vi "stateMachine.vi"() -> ()   [LabVIEW 2014]
uses:
  <vilib>/dex/Stream Element Allocation Mode.ctl
  <vilib>/Platform/TimedLoop/XDataNode/wakeup.ctl
  <vilib>/Platform/TimedLoop/XDataNode/XDNodeRunTimeDep.lvlib
  <vilib>/Platform/TimedLoop/XDataNode/nitl_modes.ctl
  <vilib>/Platform/TimedLoop/XDataNode/timing_clust.ctl
  <vilib>/platform/TimedLoop/XDataNode/XDataNode.xnode
  <resource>/objmgr/ni.dex.rc
  UDP_Para_def.ctl
  <vilib>/DAQmx/write.llb/DAQmx Write (Digital 1D Bool NChan 1Samp 1Line).vi
  states_def.ctl
  daq_channel_read_parameter.ctl
panel:
  out "rightcounter":i32
  out "leftcounter":i32
  out "beh type":string
  out "vs type":string
  out "Tab Control":enum32{"State Machine"}(tab)
  in  "vsFilterPeriod_uS":i32=500 format="%#1.6f"
  in  "lickThreshold_V":fxp<+/-,16,5> format="%#.4g"
  in  "vsThreshold_V":fxp<+/-,16,5> format="%#.4g"
  in  "audioThreshold_V":fxp<+/-,16,5> format="%#.4g"
  in  "audioFilterPeriod_uS":i32=50000 format="%#1.6f"
  in  "audioOffState_V":fxp<+/-,16,5> format="%#.4g"
  out "rtFIFOsize":u32=50
  out "rtFIFOtimeout":u32
  out "rtFIFOdataPool":u32=50
  out "stateMachineCycle_uS":i64=500
  out "(Actual)":i64
  in  "delay_uS":u32
  out "IP_RT":string="192.168.137.2"
  in  "port_broadcast":u16=9091
  out "IP_host":string="192.168.137.1"
  out "port_host":u16=9090
  in  "Tab Control 2":enum32{"Data Transfer"}(tab)
  out "stream counter":u32
  out "Is Connected":bool
  out "Available Elements for Writing":i32
  out "stream writer buffer size":i32=500
  in  "rewardPeriod_uS":u32
  in  "waterOn_uS":u32
  in  "timeout_uS":u32=5000000
  in  "shockOn_uS":u32
  in  "Stop state":bool
  out "Initial data received":bool
  out "Tab Control 3":enum32{"Current status"}(tab)
  in  "toneReward":bool
  out "ABORT":bool
  out "trialStart":bool
  out "trialDone":bool
  out "Busy":bool
  out "stateLatched":bool
  out "curKey":u32=1
  out "curState":u32
  out "rtFIFOdataDim":i32
  in  "manualShock":bool
  in  "manualWaterRight":bool
  in  "manualWaterLeft":bool
  in  "lickReward":bool
  in  "allowPunish":bool
  in  "forceLRswitch":bool
  in  "allowCorrection":bool
  in  "allowAutoWater":bool
  out "error out":errorcluster
  in  "trialKey":i32[](array[numeric])
  in  "rwdrefPeriod_uS":u32
  out "FlagWaterLeft":bool
  in  "chanellParaCluster":T1={"audioOffState_V"=0.0, "audioFilterPeriod_uS"=50000, "audioThreshold_V"=0.0, "vsThreshold_V"=0.0, "vsFilterPeriod_uS"=0, "lickThreshold_V"=0.0} {"vsFilterPeriod_uS" format="%#1.6f"; "audioFilterPeriod_uS" format="%#1.6f"}
  out "leftWaterOnFlag":bool
  out "rightWaterOnFlag":bool
  out "contNoReward":i32
  out "rewardStatus":bool
types:
  T1 = typedef "daq_channel_read_parameter.ctl" = cluster{"audioOffState_V":fxp<+/-,16,5>, "audioFilterPeriod_uS":i32, "audioThreshold_V":fxp<+/-,16,5>, "vsThreshold_V":fxp<+/-,16,5>, "vsFilterPeriod_uS":i32, "lickThreshold_V":fxp<+/-,16,5>}
  T2 = typedef "XDNodeRunTimeDep.lvlib/timing_clust.ctl" = cluster{"Expected End [f-1]":u64, "Actual End [f-1]":u64, "Finished Late? [f-1]":bool, "Expected End [i-1]":u64, "Actual End [i-1]":u64, "Finished Late? [i-1]":bool, "Expected Start [i]":u64, "Actual Start [i]":u64, "Expected Start [f]":u64, "Actual Start [f]":u64, "Source Name":string, "Structure Name":string, "Period":i64, "Deadline":i64, "Offset":i64, "Start":i64, "Priority":i32, "Timeout":i32, "Mode":T3, "Wakeup Reason":T4, "Error":errorcluster, "Source Type":string, "Secondary Source Type":string, "Global End Time":u64, "Global Start Time":u64, "Frame Duration":u64, "Iteration Duration":u64, "Assigned CPU":i32, "I/O Scan Engine Mode":u32}
  T3 = typedef "XDNodeRunTimeDep.lvlib/nitl_modes.ctl" = enum32{"No Change", "Process missed periods, maintain original phase", "Discard missed periods, maintain original phase", "Process missed periods, ignore original phase", "Discard missed periods, ignore original phase"}
  T4 = typedef "XDNodeRunTimeDep.lvlib/wakeup.ctl" = enum32{"Normal", "Aborted", "Asynchronous wakeup", "Timing source error", "Timed loop error", "Timeout"}
  T5 = typedef "states_def.ctl" = enum16{"idle", "vs before", "vs", "vs after", "delay", "tone before", "tone", "tone after", "cycle end", "reward", "reward refractory", "punish", "punish refractory", "timeout", "exit", "manualwater"}
  T6 = typedef "Stream Element Allocation Mode.ctl" = u32
  T7 = typedef "UDP_Para_def.ctl" = enum16{"no", "start", "stop", "dly", "rwp", "rwf", "wdr", "shd", "tod", "lkr", "tlr", "alp", "msh", "mwl", "mwr", "lth", "vth", "ath", "aof", "afp", "vfp"}
  T8 = cluster{"leftLick":bool, "rightLick":bool, "visualStimuli2":bool, "tone":bool, "visualStimuli1":bool}
  T9 = cluster{"leftLick":dbl, "rightLick":dbl, "visualStimuli2":dbl, "tone":dbl, "visualStimuli1":dbl}
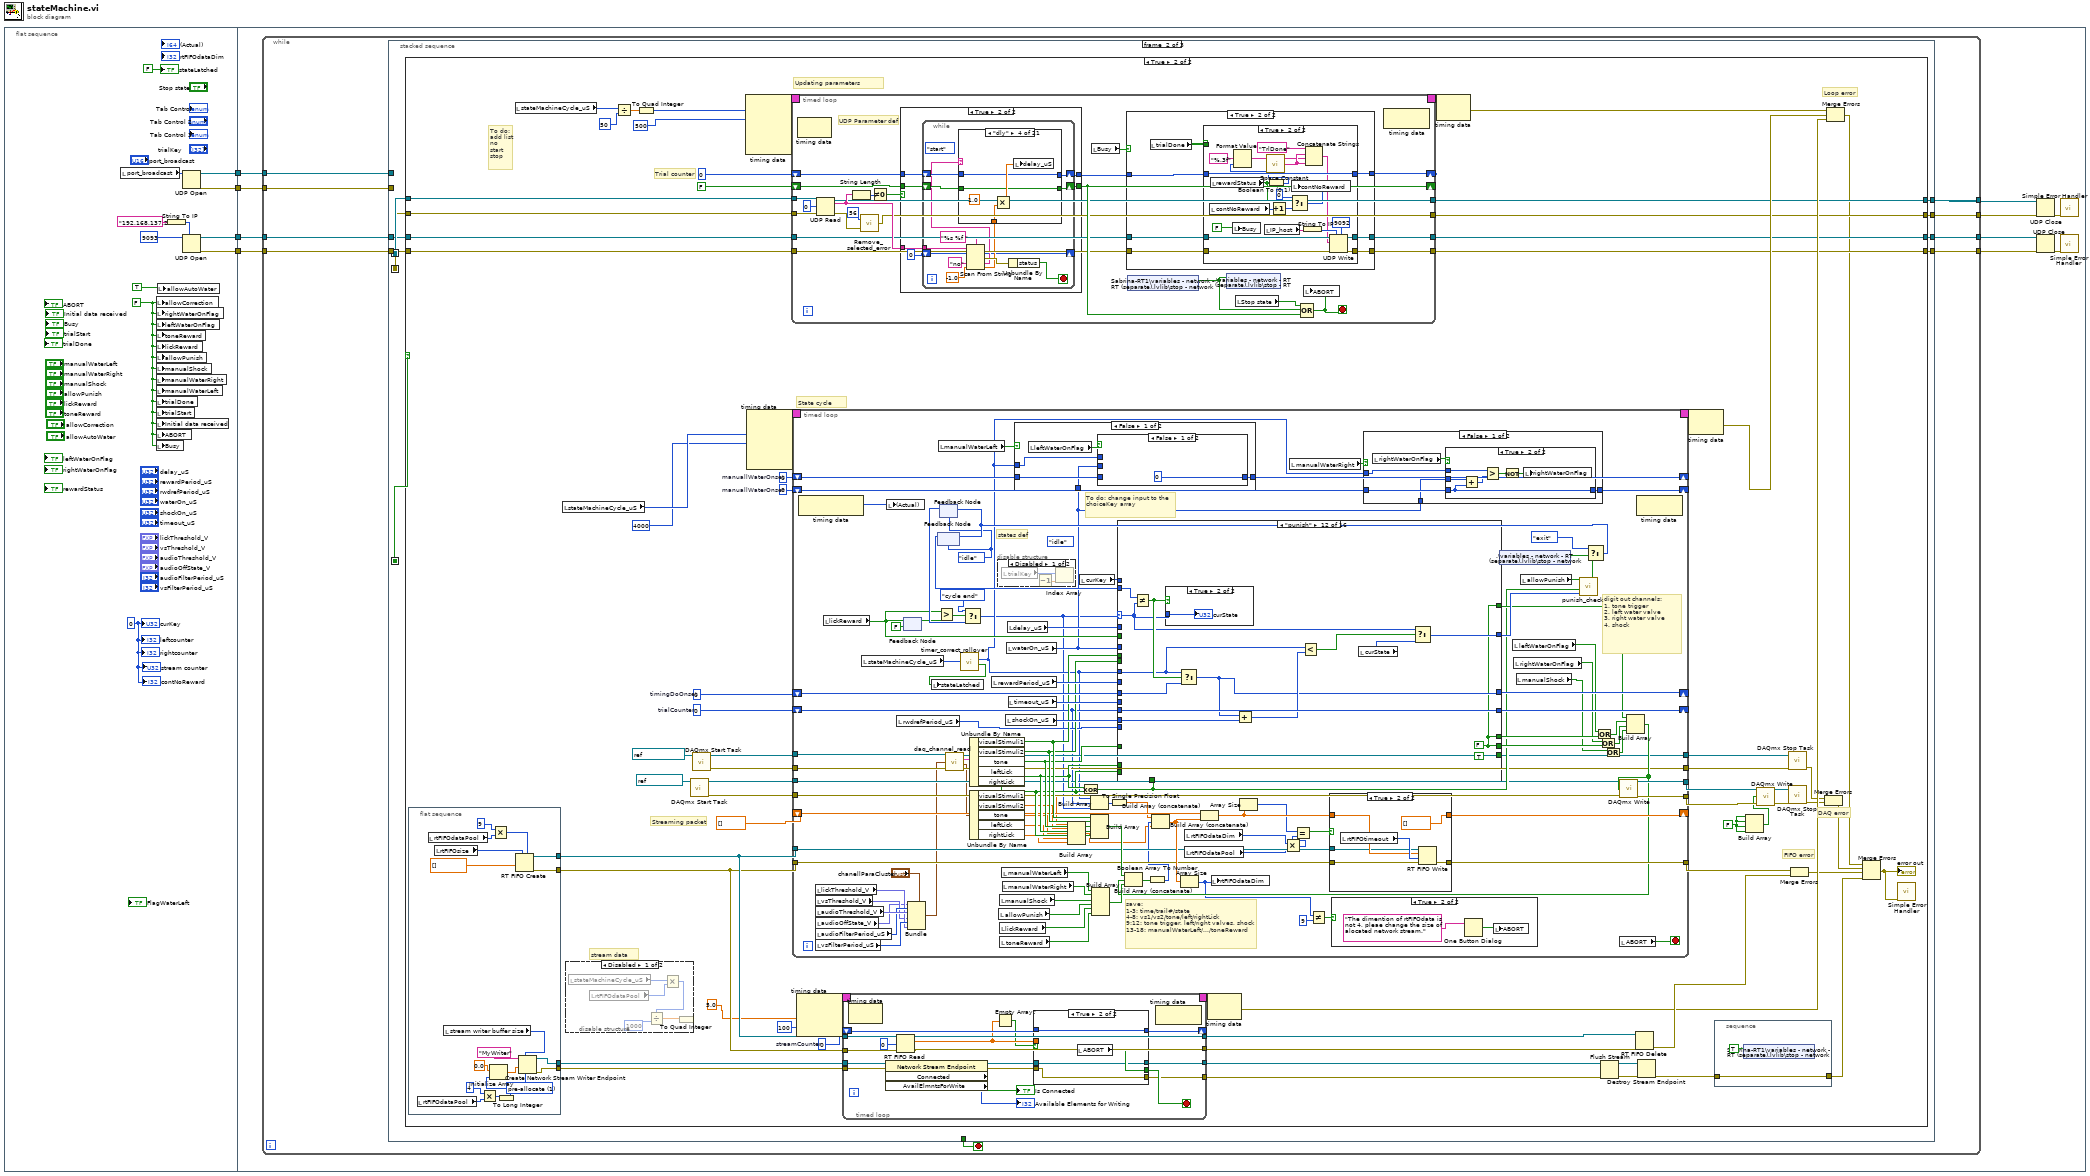
[diagram p0: block diagram]
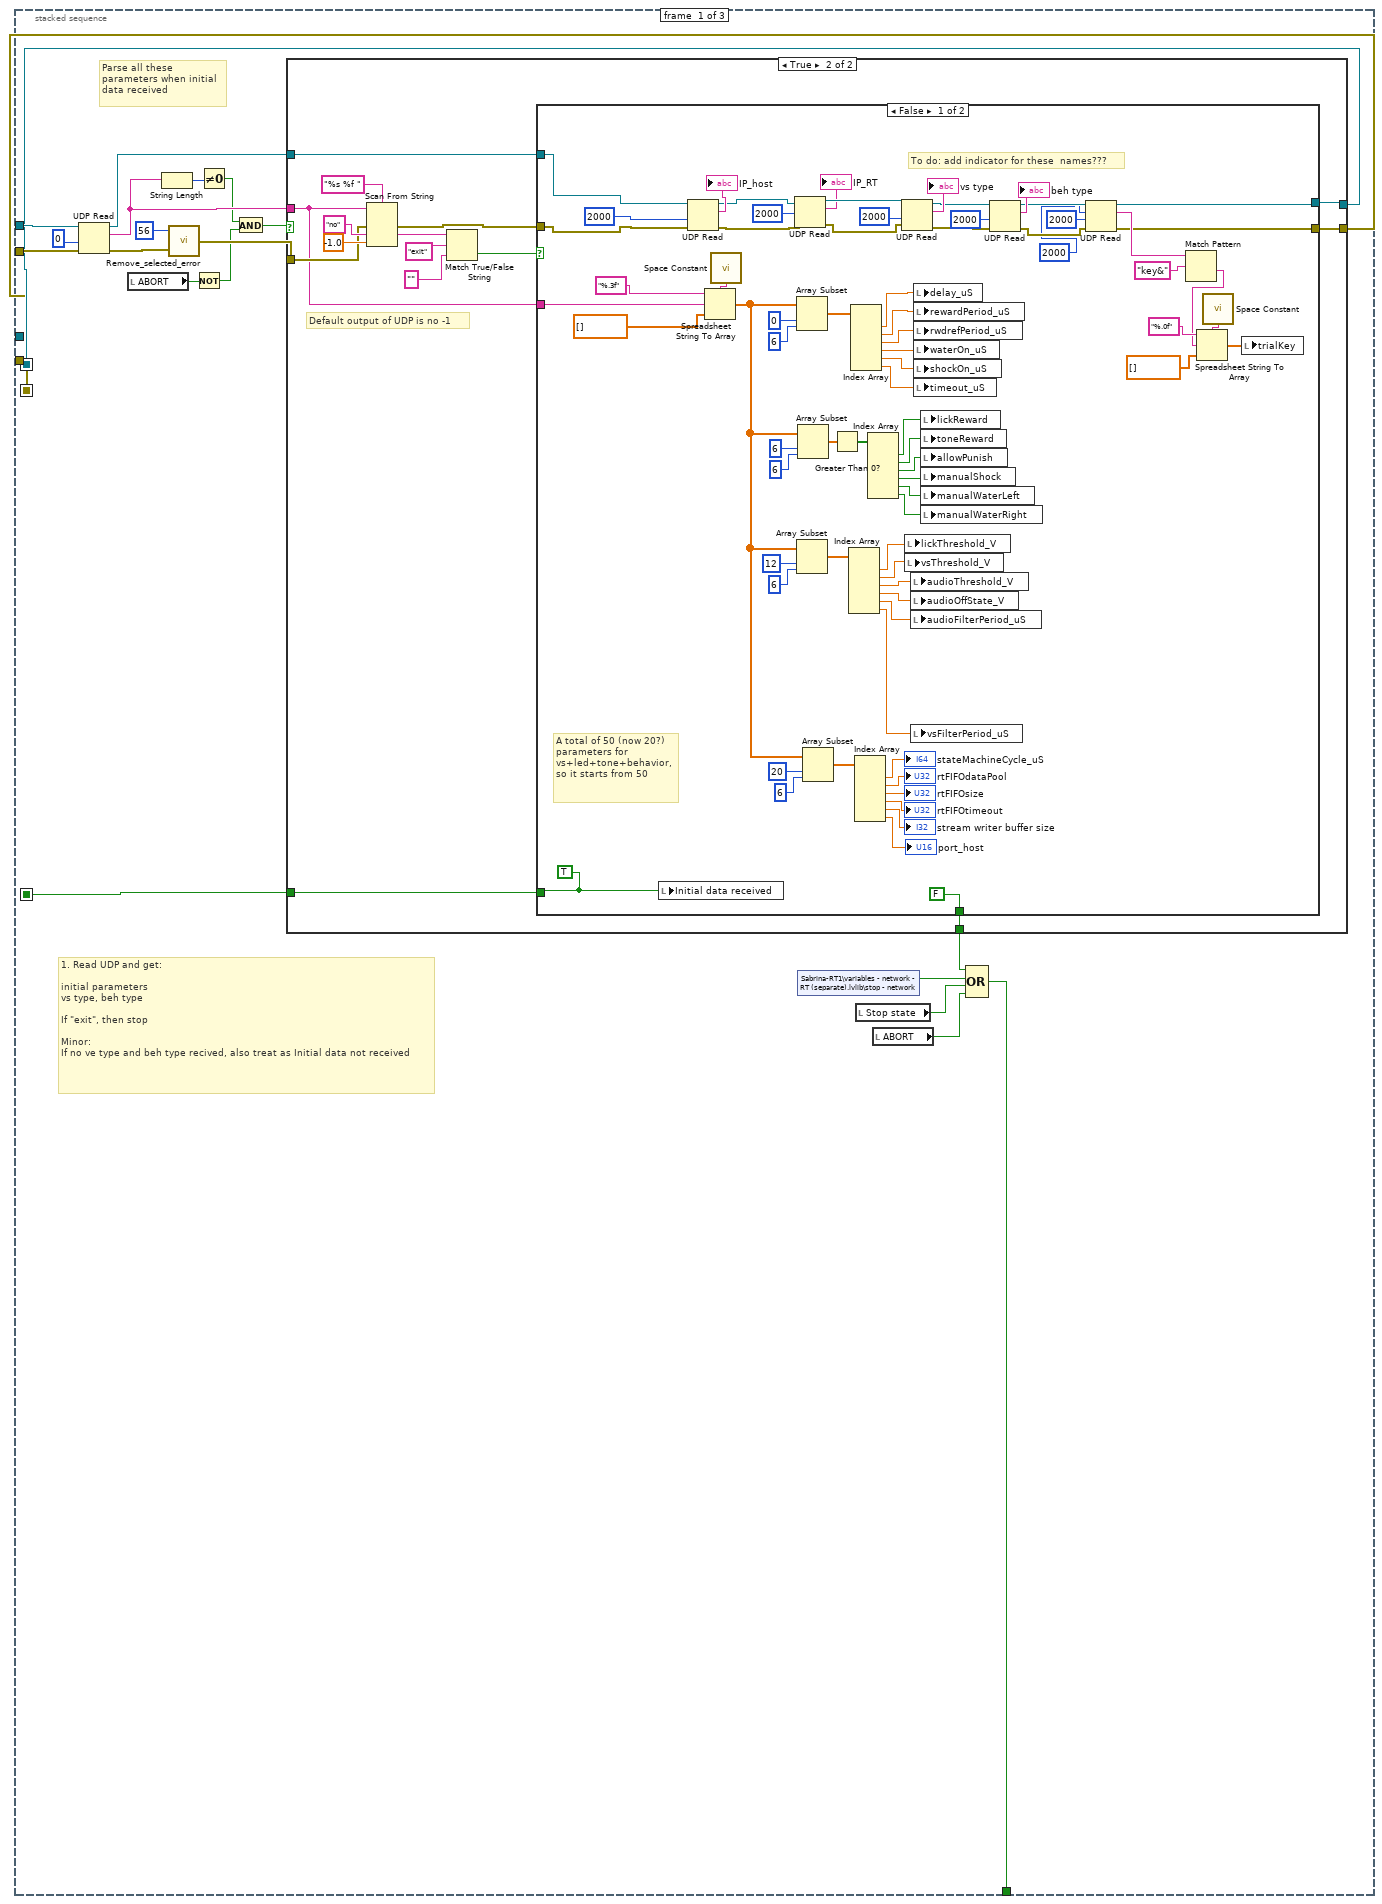
[diagram p2: hidden frame]
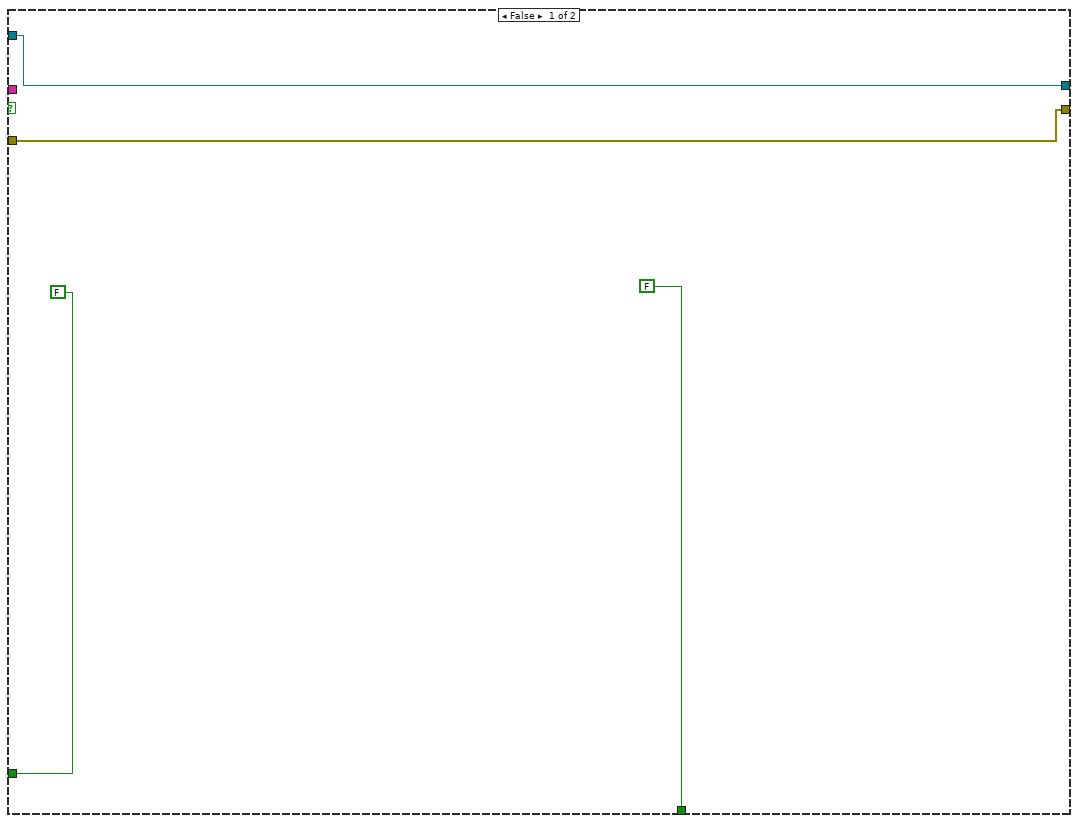
[diagram p3: hidden frame]
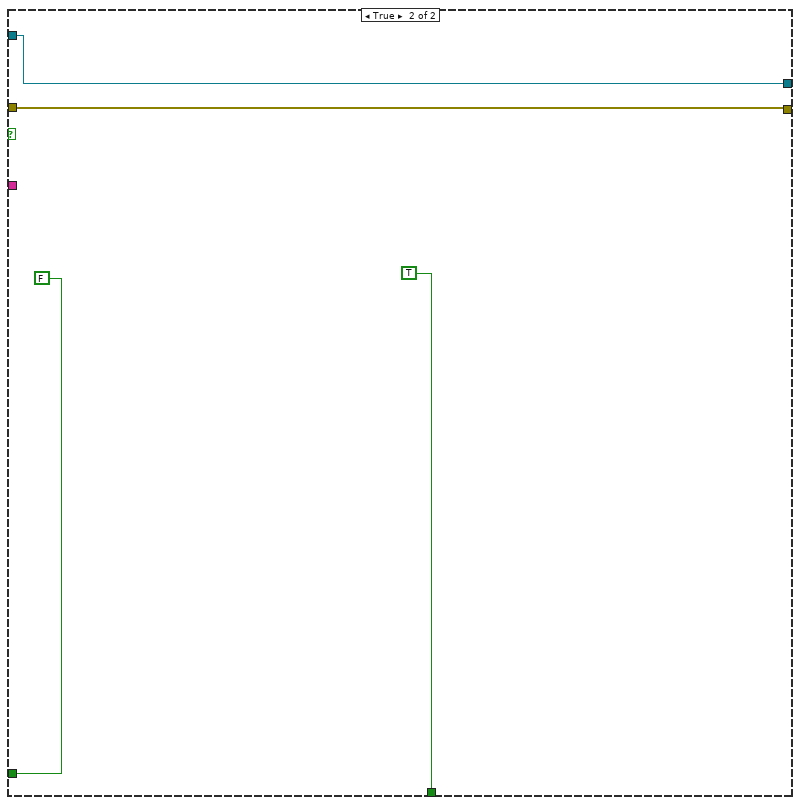
[diagram p4: hidden frame]
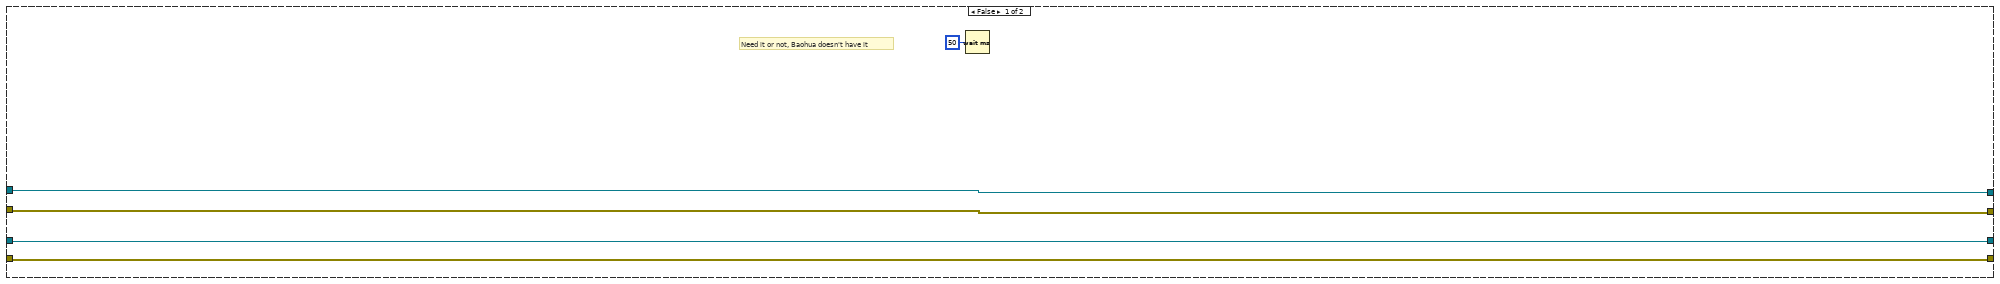
[diagram p5: hidden frame]
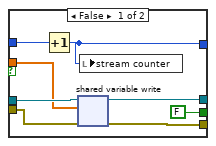
[diagram p7: hidden frame]
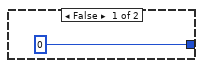
[diagram p9: hidden frame]
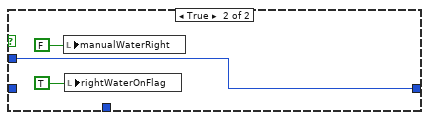
[diagram p10: hidden frame]
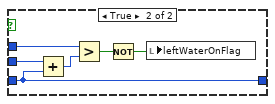
[diagram p11: hidden frame]
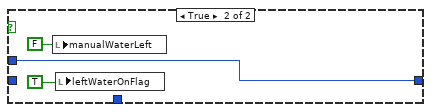
[diagram p12: hidden frame]
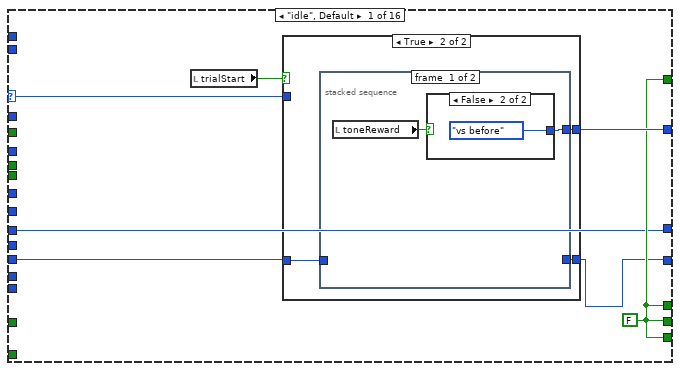
[diagram p15: hidden frame]
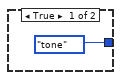
[diagram p17: hidden frame]
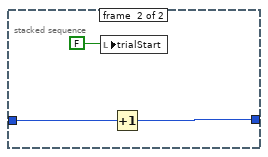
[diagram p18: hidden frame]
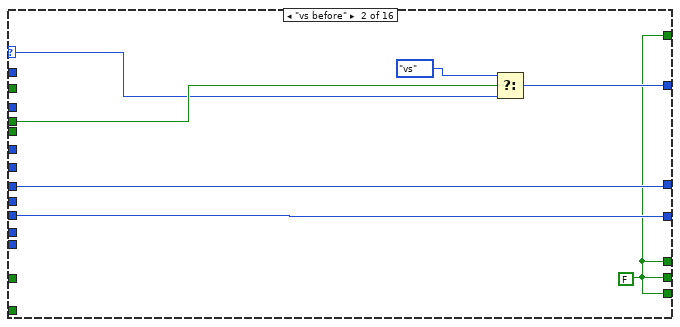
[diagram p19: hidden frame]
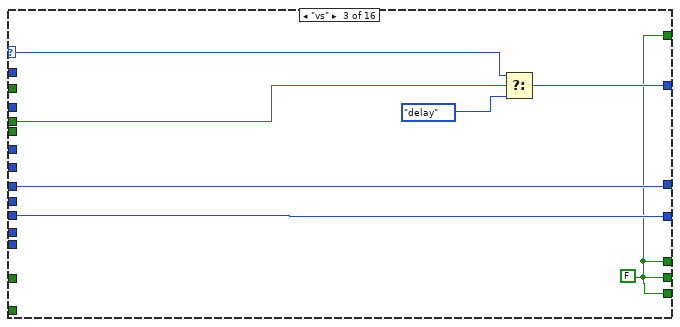
[diagram p20: hidden frame]
diagram:
  n1 = flat-sequence {
    tunnel: [w16] -> w4
    tunnel: [w15] -> w3
    tunnel: [w11] -> w2
    tunnel: [w10] -> w1
    tunnel: w4 -> [w26]
    tunnel: w3 -> [w25]
    tunnel: w2 -> [w21]
    tunnel: w1 -> [w20]
    frame #0 {
      w7 = FALSE
      w6 = 0
      n2 = local read "port_broadcast"() -> (w14:u16)
      n3 = local write "allowCorrection"(w7) -> ()
      n4 = local write "rightWaterOnFlag"(w7) -> ()
      n5 = local write "leftWaterOnFlag"(w7) -> ()
      n6 = local write "toneReward"(w7) -> ()
      n7 = local write "lickReward"(w7) -> ()
      n8 = local write "allowPunish"(w7) -> ()
      n9 = local write "manualShock"(w7) -> ()
      n10 = local write "manualWaterRight"(w7) -> ()
      n11 = local write "manualWaterLeft"(w7) -> ()
      n12 = local write "trialDone"(w7) -> ()
      n13 = local write "trialStart"(w7) -> ()
      n14 = local write "Initial data received"(w7) -> ()
      n15 = local write "ABORT"(w7) -> ()
      n16 = local write "Busy"(w7) -> ()
      n17 = local write "allowAutoWater"(TRUE) -> ()
      n18 = String To IP(1:"192.168.137.2") -> (0:w8:u32)
      n19 = UDP Open(7:w8, 11:u16 9093) -> (port=w11:refnum<k16>, 0:w10:errorcluster)  [unwired: 3 in, 1 out]
      n20 = UDP Open(11:w14) -> (port=w16:refnum<k16>, 0:w15:errorcluster)  [unwired: 4 in, 1 out]
      "stateLatched" <- FALSE
      "curKey" <- w6
      "leftcounter" <- w6
      "rightcounter" <- w6
      "stream counter" <- w6
      "contNoReward" <- w6
    }
    frame #1 {
      n21 = while {
        tunnel: w26 -> [w35]
        tunnel: w25 -> [w34]
        tunnel: [w32] -> w23
        tunnel: [w31] -> w22
        tunnel: w21 -> [w30]
        tunnel: w20 -> [w29]
        tunnel: [w28] -> w19
        tunnel: [w27] -> w18
        stop <- w33 stop-if-true
        n22 = stacked-sequence {
          seq-local: [w45 _ _] -> [_ w161 _]
          seq-local: [w37 _ _] -> [_ w158 _]
          seq-local: [w36 _ _] -> [_ w157 _]
          tunnel: w35 -> [w56 _ _]
          tunnel: w34 -> [w55 _ _]
          tunnel: [w46 _ _] -> w33
          tunnel: [_ w160 _] -> w32
          tunnel: [_ w159 _] -> w31
          tunnel: w30 -> [_ w156 _]
          tunnel: w29 -> [_ w153 _]
          tunnel: [_ w155 _] -> w28
          tunnel: [_ w154 _] -> w27
          frame #0 {
            # "Parse all these \nparameters when initial\ndata received"
            # "1. Read UDP and get:\n\ninitial parameters\nvs type, beh type\n\nIf \"exit\", then stop\n\nMinor:\nIf no ve type and beh type recived, also treat as Initial data not received"
            n23 = UDP Read(connection ID=w56, timeout ms (25000)=0, 8:w55) -> (data out=w53:string, error out=w43:errorcluster, 3:w54:refnum<k16>)  [unwired: 1 in, 2 out]
            n24 = local read "ABORT"() -> (w41:bool)
            n25 = String Length(string=w53) -> (length=w52:i32)
            n26 = call "Remove_selected_error.vi"("error in (no error)"=w43, "errorCode"=56 ("timeout ms (25000)")) -> ("error out"=w44:errorcluster)
            n27 = Not(x=w41) -> (.not. x?=w38:bool)
            n28 = Not Equal To 0?(x=w52) -> (x != 0?=w39:bool)
            n29 = And(x=w39, y=w38) -> (x .and. y?=w40:bool)
            n30 = case shown="True" w40 {
              tunnel: w53 -> [_ w65]
              tunnel: w54 -> [w58 w66]
              tunnel: w44 -> [w57 w73]
              tunnel: [FALSE w64] -> w50
              tunnel: [FALSE w63] -> w45
              tunnel: [w58 w62] -> w37
              tunnel: [w57 w61] -> w36
              frame False {
              }
              frame True {
                # "Default output of UDP is no -1"
                n31 = Scan From String(format string="%s %f ", input string=w65, error in=w73, default 1="no" ("default value 1"), default 2=sgl -1.0 ("default value 1")) -> (error out=w67:errorcluster, output 1=w72:string)  [unwired: 2 in, 2 out]
                n32 = Match True/False String(2:"" ("false string"), 3:"exit" ("true string"), 4:w72) -> (0:w68:bool)  [unwired: 1 out]
                n33 = case shown="False" w68 {
                  tunnel: w67 -> [w110 w150]
                  tunnel: w66 -> [w111 w149]
                  tunnel: w65 -> [w142 _]
                  tunnel: [FALSE TRUE] -> w64
                  tunnel: [w140 FALSE] -> w63
                  tunnel: [w77 w149] -> w62
                  tunnel: [w76 w150] -> w61
                  frame False {
                    w140 = TRUE
                    # "A total of 50 (now 20?) parameters for vs+led+tone+behavior, so it starts from 50"
                    # "To do: add indicator for these  names???"
                    n34 = local write "Initial data received"(w140) -> ()
                    n35 = UDP Read(connection ID=w111, timeout ms (25000)=2000, 8:w110) -> (data out=→"IP_host":string, error out=w109:errorcluster, 3:w107:refnum<k16>)  [unwired: 1 in, 2 out]
                    n36 = call <vilib>:"Space Constant.vi"() -> ("String"=w147:string)
                    n37 = Spreadsheet String To Array(delimiter (Tab)=w147, format string="%.3f", spreadsheet string=w142, array type (2D Dbl)=sgl[] []) -> (array=w118:sgl[])
                    n38 = UDP Read(connection ID=w107, timeout ms (25000)=2000, 8:w109) -> (data out=→"IP_RT":string, error out=w108:errorcluster, 3:w106:refnum<k16>)  [unwired: 1 in, 2 out]
                    n39 = Array Subset(array=w118, index=0 ("timeout ms (25000)"), length=6 ("timeout ms (25000)")) -> (w136:sgl[])
                    n40 = Array Subset(array=w118, index=12 ("timeout ms (25000)"), length=6 ("timeout ms (25000)")) -> (w132:sgl[])
                    n41 = Array Subset(array=w118, index=6 ("timeout ms (25000)"), length=6 ("timeout ms (25000)")) -> (w129:sgl[])
                    n42 = Array Subset(array=w118, index=20 ("timeout ms (25000)"), length=6 ("timeout ms (25000)")) -> (w119:sgl[])
                    n43 = Greater Than 0?(x=w129) -> (x > 0?=w128:bool[])
                    n44 = Index Array(array=w132) -> (element #1=w94:sgl, element #2=w93:sgl, element #3=w92:sgl, element #4=w91:sgl, element #5=w90:sgl, element #6=w89:sgl)  [unwired: 6 in]
                    n45 = Index Array(array=w136) -> (element #1=w100:sgl, element #2=w99:sgl, element #3=w98:sgl, element #4=w97:sgl, element #5=w96:sgl, element #6=w95:sgl)  [unwired: 6 in]
                    n46 = Index Array(array=w119) -> (element #1=→"stateMachineCycle_uS":sgl, element #2=→"rtFIFOdataPool":sgl, element #3=→"rtFIFOsize":sgl, element #4=→"rtFIFOtimeout":sgl, element #5=→"stream writer buffer size":sgl, element #6=→"port_host":sgl)  [unwired: 6 in]
                    n47 = Index Array(array=w128) -> (element #1=w127:bool, element #2=w126:bool, element #3=w125:bool, element #4=w124:bool, element #5=w123:bool, element #6=w122:bool)  [unwired: 6 in]
                    n48 = UDP Read(connection ID=w106, timeout ms (25000)=2000, 8:w108) -> (data out=→"vs type":string, error out=w139:errorcluster, 3:w138:refnum<k16>)  [unwired: 1 in, 2 out]
                    n49 = local write "lickThreshold_V"(w94) -> ()
                    n50 = local write "vsThreshold_V"(w93) -> ()
                    n51 = local write "audioThreshold_V"(w92) -> ()
                    n52 = local write "audioOffState_V"(w91) -> ()
                    n53 = local write "audioFilterPeriod_uS"(w90) -> ()
                    n54 = local write "vsFilterPeriod_uS"(w89) -> ()
                    n55 = local write "delay_uS"(w100) -> ()
                    n56 = local write "rewardPeriod_uS"(w99) -> ()
                    n57 = local write "rwdrefPeriod_uS"(w98) -> ()
                    n58 = local write "waterOn_uS"(w97) -> ()
                    n59 = local write "shockOn_uS"(w96) -> ()
                    n60 = local write "timeout_uS"(w95) -> ()
                    n61 = local write "lickReward"(w127) -> ()
                    n62 = local write "toneReward"(w126) -> ()
                    n63 = local write "allowPunish"(w125) -> ()
                    n64 = local write "manualShock"(w124) -> ()
                    n65 = local write "manualWaterLeft"(w123) -> ()
                    n66 = local write "manualWaterRight"(w122) -> ()
                    n67 = UDP Read(connection ID=w138, timeout ms (25000)=2000, 8:w139) -> (data out=→"beh type":string, error out=w86:errorcluster, 3:w87:refnum<k16>)  [unwired: 1 in, 2 out]
                    n68 = UDP Read(connection ID=w87, max size (548)=2000 ("timeout ms (25000)"), timeout ms (25000)=2000, 8:w86) -> (data out=w81:string, error out=w76:errorcluster, 3:w77:refnum<k16>)  [unwired: 2 out]
                    n69 = Match Pattern(string=w81, regular expression="key&") -> (after substring=w79:string)  [unwired: 1 in, 3 out]
                    n70 = call <vilib>:"Space Constant.vi"() -> ("String"=w84:string)
                    n71 = Spreadsheet String To Array(delimiter (Tab)=w84, format string="%.0f", spreadsheet string=w79, array type (2D Dbl)=dbl[] []) -> (array=w82:dbl[])
                    n72 = local write "trialKey"(w82) -> ()
                  }
                  frame True {
                  }
                }
              }
            }
            n73 = shared-variable "Sabrina-RT1\\variables - network - RT (separate).lvlib\\stop - network"() -> (w49:bool)  [unwired: 1 in, 1 out]
            n74 = local read "Stop state"() -> (w48:bool)
            n75 = local read "ABORT"() -> (w47:bool)
            n76 = Compound Arithmetic op=OR(w50, w49, w48, w47) -> (w46:bool)
          }
          frame #1 {
            n77 = case shown="True" w161 {
              tunnel: w158 -> [w165 w211]
              tunnel: w157 -> [w164 w210]
              tunnel: [w165 w183] -> w160
              tunnel: [w164 w184] -> w159
              tunnel: w156 -> [w163 w188]
              tunnel: w153 -> [w162 w187]
              tunnel: [w162 w186] -> w155
              tunnel: [w163 w185] -> w154
              frame False {
                # "Need it or not, Baohua doesn't have it"
                n78 = Wait (ms)(milliseconds to wait=u32 50) -> ()  [unwired: 1 out]
              }
              frame True {
                w167 = 0  # manuallWaterOnset
                w168 = 0  # manuallWaterOnset
                w194 = FALSE
                w223 = 0  # streamCounter
                w226 = 0  # timingDoOnset
                w225 = 0  # trialCounter
                # "Streaming packet"
                # "Trial counter"
                # "Loop error"
                # "DAQ error"
                # "FIFO error"
                # "Updating parameters"
                # "State cycle"
                # "To do:\nadd list\nno\nstart\nstop"
                # "stream data"
                n79 = flat-sequence {
                  tunnel: [w253] -> w228
                  tunnel: [w252] -> w227
                  tunnel: [w251] -> w214
                  tunnel: [w250] -> w213
                  frame #0 {
                    w257 = T6 1 items=["allocate as needed", "pre-allocate"] ("element allocation mode")
                    n80 = local read "rtFIFOdataPool"() -> (w248:u32)
                    n81 = local read "rtFIFOdataPool"() -> (w245:u32)
                    n82 = local read "rtFIFOsize"() -> (w259:u32)
                    n83 = local read "stream writer buffer size"() -> (w249:i32)
                    n84 = Multiply(x=u32 4, y=w248) -> (x*y=w243:u32)
                    n85 = Multiply(x=9, y=w245) -> (x*y=w244:u32)
                    n86 = To Long Integer(number=w243) -> (32bit integer=w242:i32)
                    n87 = Initialize Array(sgl 0.0, w242) -> (w256:sgl[])
                    n88 = RT FIFO Create(1:sgl[] [], 4:w259, 6:w244) -> (8:w251:refnum<k33>, 11:w250:errorcluster)  [unwired: 5 in, 1 out]
                    n89 = Create Network Stream Writer Endpoint(6:w257, 7:w249, 9:w256, 11:"MyWriter" ("writer name")) -> (0:w253:errorcluster, 3:w252:refnum<k21>)  [unwired: 3 in]
                  }
                }
                n90 = local read "stateMachineCycle_uS"() -> (w212:i64)
                n91 = local read "stateMachineCycle_uS"() -> (w222:i64)
                n92 = disable-structure shown="Disabled" {
                  frame Disabled {
                    n93 = local read "stateMachineCycle_uS"() -> (w237:i64)
                    n94 = local read "rtFIFOdataPool"() -> (w236:u32)
                    n95 = Multiply(x=w237, y=w236) -> (x*y=w238:i64)
                    n96 = Divide(x=w238, y=i64 1000) -> (x/y=w235:dbl)
                    n97 = To Quad Integer(1:w235) -> ()  [unwired: 1 out]
                  }
                  frame Enabled {
                  }
                }
                n98 = Divide(x=w212, y=i64 50) -> (x/y=w218:dbl)
                n99 = To Quad Integer(1:w218) -> (0:w217:i64)
                n100 = call <vilib>:"DAQmx Start Task.vi"("task/channels in"=refnum<k21> "digitWrite" ("digitWrite")) -> ("task out"=w180:refnum<k21>, "error out"=w179:errorcluster)  [unwired: 13 in]
                n101 = call <vilib>:"DAQmx Start Task.vi"("task/channels in"=refnum<k21> "analogRead" ("DAQmx Task Name")) -> ("task out"=w170:refnum<k21>, "error out"=w169:errorcluster)  [unwired: 13 in]
                n102 = node-c288(w217, 500 ("Priority")) -> (w234:T2)  [unwired: 3 in]
                n103 = node-c288(w222, 4000 ("Priority")) -> (w232:T2)  [unwired: 3 in]
                n104 = timed-loop {
                  timing: w234 -> [_]
                  timing-out: [_] -> w233
                  shift-right: [w735] -> _
                  shift-left: 0 ("timeout ms (25000)") -> [w737]
                  shift-right: [w731] -> _
                  shift-left: FALSE -> [w734]
                  tunnel: [w728] -> w185
                  tunnel: [w727] -> w186
                  tunnel: w211 -> [w726]
                  tunnel: w210 -> [w725]
                  tunnel: w188 -> [w719]
                  tunnel: w187 -> [w722]
                  tunnel: [w721] -> w184
                  tunnel: [w720] -> w183
                  stop <- w733 stop-if-true
                  # "UDP Parameter def"
                  n105 = node-c288() -> ()  [unwired: 1 in, 1 out]
                  n106 = UDP Read(connection ID=w726, timeout ms (25000)=0, 8:w725) -> (data out=w738:string, error out=w724:errorcluster, 3:w720:refnum<k16>)  [unwired: 1 in, 2 out]
                  n107 = String Length(string=w738) -> (length=w740:i32)
                  n108 = call "Remove_selected_error.vi"("error in (no error)"=w724, "errorCode"=56 ("timeout ms (25000)")) -> ("error out"=w721:errorcluster)
                  n109 = Not Equal To 0?(x=w740) -> (x != 0?=w739:bool)
                  n110 = case shown="True" w739 {
                    tunnel: w738 -> [_ w782]
                    tunnel: w737 -> [w776 w781]
                    tunnel: [w776 w780] -> w736
                    tunnel: w734 -> [w775 w779]
                    tunnel: [w775 w778] -> w731
                    frame False {
                    }
                    frame True {
                      n111 = while {
                        tunnel: w782 -> [w796]
                        shift-right: [w783] -> _
                        shift-left: 0 ("timeout ms (25000)") -> [w784]
                        shift-right: [w789] -> w780
                        shift-left: w781 -> [w790]
                        shift-right: [w787] -> w778
                        shift-left: w779 -> [w788]
                        stop <- w791 stop-if-true
                        (unwired) UDP_Para_def."start"
                        n112 = Scan From String(format string="%s %f ", input string=w796, initial scan location=w784, default 1="no" ("default value 1"), default 2=-1.0 ("default value 2")) -> (offset past scan=w783:u32, error out=w792:errorcluster, output 1=w786:string, output 2=w785:dbl)  [unwired: 1 in, 1 out]
                        n113 = case shown="\"dly\"" w786 {
                          tunnel: [w798 w800 w809 w811 w816 w821 w826 w831 w836 w841 w845 w849 w853 w857 w861 w865 w869 w873 w877 w881 w886] -> w789
                          tunnel: w790 -> [w798 w801 w809 w811 w816 w821 w826 w831 w836 w841 w845 w849 w853 w857 w861 w865 w869 w873 w877 w881 w886]
                          tunnel: [w797 w805 w806 w810 w815 w820 w825 w830 w835 w840 w844 w848 w852 w856 w860 w864 w868 w872 w876 w880 w885] -> w787
                          tunnel: w788 -> [w797 w805 w807 w810 w815 w820 w825 w830 w835 w840 w844 w848 w852 w856 w860 w864 w868 w872 w876 w880 w885]
                          tunnel: w785 -> [_ w802 _ w813 w818 w823 w828 w833 w838 w843 w847 w851 w855 w859 w863 w867 w871 w875 w879 w883 w888]
                          frame "no", Default {
                          }
                          frame "start" {
                            w804 = TRUE
                            n114 = Increment(x=w801) -> (x+1=w800:i32)
                            n115 = local write "rewardStatus"(FALSE) -> ()
                            n116 = local write "trialDone"(FALSE) -> ()
                            n117 = local write "Busy"(w804) -> ()
                            n118 = local write "trialStart"(w804) -> ()
                            n119 = local write "curKey"(w802) -> ()
                          }
                          frame "stop" {
                            n120 = Or(x=w807, y=TRUE) -> (x .or. y?=w806:bool)
                          }
                          frame "dly" {
                            n121 = Multiply(x=1.0, y=w813) -> (x*y=w812:dbl)
                            n122 = local write "delay_uS"(w812) -> ()
                          }
                          frame "rwp" {
                            n123 = Multiply(x=1.0, y=w818) -> (x*y=w817:dbl)
                            n124 = local write "rewardPeriod_uS"(w817) -> ()
                          }
                          frame "rwf" {
                            n125 = Multiply(x=1.0, y=w823) -> (x*y=w822:dbl)
                            n126 = local write "rwdrefPeriod_uS"(w822) -> ()
                          }
                          frame "wdr" {
                            n127 = Multiply(x=1.0, y=w828) -> (x*y=w827:dbl)
                            n128 = local write "waterOn_uS"(w827) -> ()
                          }
                          frame "shd" {
                            n129 = Multiply(x=1.0, y=w833) -> (x*y=w832:dbl)
                            n130 = local write "shockOn_uS"(w832) -> ()
                          }
                          frame "tod" {
                            n131 = Multiply(x=1.0, y=w838) -> (x*y=w837:dbl)
                            n132 = local write "timeout_uS"(w837) -> ()
                          }
                          frame "lkr" {
                            n133 = Greater Than 0?(x=w843) -> (x > 0?=w842:bool)
                            n134 = local write "lickReward"(w842) -> ()
                          }
                          frame "tlr" {
                            n135 = Greater Than 0?(x=w847) -> (x > 0?=w846:bool)
                            n136 = local write "toneReward"(w846) -> ()
                          }
                          frame "alp" {
                            n137 = Greater Than 0?(x=w851) -> (x > 0?=w850:bool)
                            n138 = local write "allowPunish"(w850) -> ()
                          }
                          frame "msh" {
                            n139 = Greater Than 0?(x=w855) -> (x > 0?=w854:bool)
                            n140 = local write "manualShock"(w854) -> ()
                          }
                          frame "mwl" {
                            n141 = Greater Than 0?(x=w859) -> (x > 0?=w858:bool)
                            n142 = local write "manualWaterLeft"(w858) -> ()
                          }
                          frame "mwr" {
                            n143 = Greater Than 0?(x=w863) -> (x > 0?=w862:bool)
                            n144 = local write "manualWaterRight"(w862) -> ()
                          }
                          frame "lth" {
                            n145 = To Fixed-Point(number=w867) -> (fixed-point=w866:fxp<+/-,32,16>)  [unwired: 1 in]
                            n146 = local write "lickThreshold_V"(w866) -> ()
                          }
                          frame "vth" {
                            n147 = To Fixed-Point(number=w871) -> (fixed-point=w870:fxp<+/-,32,16>)  [unwired: 1 in]
                            n148 = local write "vsThreshold_V"(w870) -> ()
                          }
                          frame "ath" {
                            n149 = To Fixed-Point(number=w875) -> (fixed-point=w874:fxp<+/-,32,16>)  [unwired: 1 in]
                            n150 = local write "audioThreshold_V"(w874) -> ()
                          }
                          frame "aof" {
                            n151 = To Fixed-Point(number=w879) -> (fixed-point=w878:fxp<+/-,32,16>)  [unwired: 1 in]
                            n152 = local write "audioOffState_V"(w878) -> ()
                          }
                          frame "afp" {
                            n153 = Multiply(x=1.0, y=w883) -> (x*y=w882:dbl)
                            n154 = local write "audioFilterPeriod_uS"(w882) -> ()
                          }
                          frame "vfp" {
                            n155 = Multiply(x=1.0, y=w888) -> (x*y=w887:dbl)
                            n156 = local write "vsFilterPeriod_uS"(w887) -> ()
                          }
                        }
                        n157 = Unbundle By Name(w792) -> ("status"=w791:bool)
                      }
                    }
                  }
                  n158 = local read "Busy"() -> (w732:bool)
                  n159 = case shown="True" w732 {
                    tunnel: w736 -> [w744 w751]
                    tunnel: [w744 w750] -> w735
                    tunnel: w719 -> [w743 w749]
                    tunnel: [w743 w748] -> w728
                    tunnel: [w742 w747] -> w727
                    tunnel: w722 -> [w742 w746]
                    frame False {
                    }
                    frame True {
                      n160 = local read "trialDone"() -> (w745:bool)
                      n161 = case shown="True" w745 {
                        tunnel: w751 -> [w754 w769]
                        tunnel: [w754 w769] -> w750
                        tunnel: w749 -> [w753 w768]
                        tunnel: [w753 w767] -> w748
                        tunnel: [w752 w766] -> w747
                        tunnel: w745 -> [_ _]
                        tunnel: w746 -> [w752 w763]
                        frame False {
                        }
                        frame True {
                          n162 = local read "contNoReward"() -> (w757:i32)
                          n163 = local read "rewardStatus"() -> (w759:bool)
                          n164 = local write "Busy"(FALSE) -> ()
                          n165 = local read "IP_host"() -> (w764:string)
                          n166 = call <vilib>:"Space Constant.vi"() -> ("String"=w773:string)
                          n167 = Boolean To (0,1)(Boolean=w759) -> (0, 1=w760:i16)
                          n168 = Format Value(format string="%.3f", value (0)=w760) -> (output string=w771:string)  [unwired: 1 in]
                          n169 = Increment(x=w757) -> (x+1=w756:i32)
                          n170 = Select(t=0 ("timeout ms (25000)"), s=w759, f=w756) -> (s? t:f=w755:i32)
                          n171 = local write "contNoReward"(w755) -> ()
                          n172 = String To IP(1:w764) -> (0:w770:u32)
                          n173 = Concatenate Strings("TrlDone" ("data in"), w773, w771, w773) -> (w762:string)
                          n174 = UDP Write(address=w770, port or service name=u16 9092, connection ID=w768, data in=w762, 8:w763) -> (error out=w766:errorcluster, 3:w767:refnum<k16>)  [unwired: 1 in]
                        }
                      }
                    }
                  }
                  n175 = shared-variable "Sabrina-RT1\\variables - network - RT (separate).lvlib\\stop - network"() -> (w730:bool)  [unwired: 1 in, 1 out]
                  n176 = shared-variable ".\\variables - network - RT (separate).lvlib\\stop - RT"(w730) -> ()  [unwired: 1 in, 1 out]
                  n177 = local read "Stop state"() -> (w729:bool)
                  n178 = Compound Arithmetic op=OR(w729, w730, w731) -> (w733:bool)
                  n179 = local write "ABORT"(w733) -> ()
                  n180 = node-c288() -> ()  [unwired: 1 in, 1 out]
                }
                n181 = timed-loop {
                  timing: w232 -> [_]
                  timing-out: [_] -> w231
                  shift-right: [w383] -> _
                  shift-left: w225 -> [w318]
                  tunnel: [w396] -> w201
                  tunnel: [w395] -> w200
                  shift-right: [w393] -> _
                  shift-left: w226 -> [w394]
                  tunnel: w170 -> [w385]
                  tunnel: w169 -> [w348]
                  tunnel: [w320] -> w175
                  shift-right: [w376] -> _
                  shift-left: sgl[] [] ("array type (2D Dbl)") -> [w377]
                  tunnel: [w373] -> w191
                  tunnel: w214 -> [w347]
                  tunnel: w213 -> [w346]
                  tunnel: w180 -> [w336]
                  tunnel: w179 -> [w335]
                  tunnel: [w330] -> w176
                  shift-right: [w308] -> _
                  shift-left: w168 -> [w309]
                  shift-right: [w304] -> _
                  shift-left: w167 -> [w305]
                  stop <- w331 stop-if-true
                  w340 = states_def."idle"
                  (unwired) states_def."idle"
                  # "states def"
                  # "save: \n1-3: time/trail#/state\n4-8: vs1/vs2/tone/left/rightLick\n9:12: tone trigger, left/right valves, shock\n13-18: manualWaterLeft/.../toneReward"
                  # "digit out channels:\n1. tone trigger\n2. left water valve\n3. right water valve\n4. shock"
                  # "To do: change input to the choiceKey array"
                  n182 = node-c288() -> (w343:i64)  [unwired: 1 in]
                  n183 = local read "lickThreshold_V"() -> (w324:fxp<+/-,16,5>)
                  n184 = local read "vsThreshold_V"() -> (w323:fxp<+/-,16,5>)
                  n185 = local read "audioThreshold_V"() -> (w329:fxp<+/-,16,5>)
                  n186 = local read "audioOffState_V"() -> (w322:fxp<+/-,16,5>)
                  n187 = local read "audioFilterPeriod_uS"() -> (w325:i32)
                  n188 = local read "vsFilterPeriod_uS"() -> (w326:i32)
                  n189 = local read "lickReward"() -> (w349:bool)
                  n190 = local read "stateMachineCycle_uS"() -> (w344:i64)
                  n191 = local write "(Actual)"(w343) -> ()
                  n192 = local read "rwdrefPeriod_uS"() -> (w337:u32)
                  n193 = feedback #1(FALSE ("lick-reward")) -> (w399:bool)
                  n194 = feedback-in #1(w349) -> ()
                  n195 = Bundle(cluster="chanellParaCluster", "audioOffState_V"=w322, "audioFilterPeriod_uS"=w325, "audioThreshold_V"=w329, "vsThreshold_V"=w323, "vsFilterPeriod_uS"=w326, "lickThreshold_V"=w324) -> (w328:T1)
                  n196 = feedback #2(w340) -> (w397:T5)
                  n197 = Greater?(x=w349, y=w399) -> (0:w400:bool)
                  n198 = local read "manualWaterLeft"() -> (w310:bool)
                  n199 = feedback #3(w340) -> (w401:T5)
                  n200 = call "daq_channel_read.vi"("DAQmxTaskIn"=w385, "chanellParaCluster"=w328, "error in (no error)"=w348) -> ("DAQmxTaskOut"=w330:refnum<k21>, "channelOutCluster"=w321:T8, "channelOutCluster_rawData"=w319:T9, "error out"=w320:errorcluster)
                  n201 = call "timer_correct_rollover.vi"("Loop Rate(uSec)"=w344) -> ("Late? (Latched)"=w386:bool, "Tick Count(uSec)"=w303:u64)  [unwired: 8 in, 1 out]
                  n202 = local write "stateLatched"(w386) -> ()
                  n203 = Select(t=states_def."cycle end", s=w400, f=w401) -> (s? t:f=w299:T5)
                  n204 = Unbundle By Name(w321) -> ("visualStimuli1"=w382:bool, "visualStimuli2"=w381:bool, "tone"=w380:bool, "leftLick"=w379:bool, "rightLick"=w378:bool)
                  n205 = Unbundle By Name(w319) -> ("visualStimuli1"=w312:dbl, "visualStimuli2"=w317:dbl, "tone"=w316:dbl, "leftLick"=w315:dbl, "rightLick"=w314:dbl)
                  n206 = local read "rewardPeriod_uS"() -> (w389:u32)
                  n207 = disable-structure shown="Disabled" {
                    frame Disabled {
                      n208 = local read "trialKey"() -> (w404:i32[])
                      n209 = Decrement() -> (x-1=w403:dbl)  [unwired: 1 in]
                      n210 = Index Array(array=w404, index=w403) -> ()  [unwired: 1 out]
                    }
                    frame Enabled {
                    }
                  }
                  n211 = local read "allowPunish"() -> (w360:bool)
                  n212 = local read "manualShock"() -> (w359:bool)
                  n213 = local read "lickReward"() -> (w361:bool)
                  n214 = local read "toneReward"() -> (w338:bool)
                  n215 = local read "manualWaterLeft"() -> (w358:bool)
                  n216 = local read "manualWaterRight"() -> (w357:bool)
                  n217 = local read "shockOn_uS"() -> (w384:u32)
                  n218 = local read "waterOn_uS"() -> (w302:u32)
                  n219 = local read "delay_uS"() -> (w339:u32)
                  n220 = local read "timeout_uS"() -> (w388:u32)
                  n221 = case shown="False" w310 {
                    tunnel: w309 -> [w423 _]
                    tunnel: [w422 w434] -> w308
                    tunnel: w303 -> [w421 w434]
                    tunnel: w302 -> [w420 _]
                    frame False {
                      n222 = local read "leftWaterOnFlag"() -> (w424:bool)
                      n223 = case shown="False" w424 {
                        tunnel: w423 -> [_ w429]
                        tunnel: [0 w429] -> w422
                        tunnel: w421 -> [_ w431]
                        tunnel: w420 -> [_ w430]
                        frame False {
                        }
                        frame True {
                          n224 = Add(x=w430, y=w429) -> (x+y=w428:u64)
                          n225 = Greater?(x=w431, y=w428) -> (0:w427:bool)
                          n226 = Not(x=w427) -> (.not. x?=w426:bool)
                          n227 = local write "leftWaterOnFlag"(w426) -> ()
                        }
                      }
                    }
                    frame True {
                      n228 = local write "manualWaterLeft"(FALSE) -> ()
                      n229 = local write "leftWaterOnFlag"(TRUE) -> ()
                    }
                  }
                  n230 = Build Array(w312, w317, w316, w315, w314) -> (w311:dbl[])
                  n231 = local read "curKey"() -> (w300:u32)
                  n232 = Exclusive Or(1:w378, 2:w379) -> (0:w366:bool)
                  n233 = Build Array(w303, w318, w299) -> (w355:u64[])
                  n234 = Build Array(w382, w381, w380, w379, w378) -> (w365:bool[])
                  n235 = Build Array(w358, w357, w359, w360, w361, w338) -> (w364:bool[])
                  n236 = To Single Precision Float(number=w355) -> (single precision float=w356:sgl[])
                  n237 = case shown="\"punish\"" w299 {
                    selector: w299 -> [w448 w468 w476 w484 w490 w506 w519 w528 w607 w626 w661 w669 w683 w694 w700 _]
                    tunnel: w382 -> [_ w470 w477 w483 _ _ _ _ _ _ _ _ _ _ _ _]
                    tunnel: w397 -> [_ _ _ _ w491 _ _ _ _ w644 _ w675 _ w695 _ _]
                    tunnel: w303 -> [_ _ _ _ w493 w501 w515 w543 w610 w642 w658 w670 _ w692 _ _]
                    tunnel: [w451 w469 w475 w482 w497 w500 w520 w542 w614 w640 w662 w673 w683 w693 w700 states_def."tone after"] -> w392
                    tunnel: w381 -> [_ _ _ _ _ _ _ _ _ _ _ _ _ _ _ _]
                    tunnel: [w449 w464 w471 w478 w487 w499 w517 w534 w611 w632 w666 w667 w682 w686 w699 w703] -> w371
                    tunnel: w349 -> [_ _ _ _ _ _ _ w532 w615 w629 _ _ _ _ _ _]
                    tunnel: w318 -> [w445 w466 w473 w480 w496 w502 w518 w537 w613 w636 w659 w679 w684 w688 w702 w704]
                    tunnel: w380 -> [_ _ _ _ _ w504 _ _ _ _ _ _ _ _ _ _]
                    tunnel: w394 -> [w447 w467 w474 w481 w486 w505 w514 w538 w609 w634 w664 w678 w685 w691 w701 w705]
                    tunnel: [w447 w467 w474 w481 w488 w503 w516 w538 w608 w633 w655 w671 w685 w689 w701 w705] -> w393
                    tunnel: w379 -> [_ _ _ _ _ _ _ w540 _ _ _ _ _ _ _ _]
                    tunnel: w378 -> [_ _ _ _ _ _ _ w539 _ _ _ _ _ _ _ _]
                    tunnel: [w449 w464 w471 w478 w487 w498 w517 w534 w611 w638 w666 w667 w682 w686 w699 w703] -> w370
                    tunnel: [w449 w464 w471 w478 w487 w498 w517 w534 w611 w637 w666 w667 w682 w686 w699 w703] -> w368
                    tunnel: [w446 w466 w473 w480 w496 w502 w518 w537 w612 w636 w659 w679 w684 w688 w702 w704] -> w383
                    tunnel: w366 -> [_ _ _ _ _ _ _ w536 _ _ _ _ _ _ _ _]
                    tunnel: w389 -> [_ _ _ _ _ _ _ w535 _ _ _ _ _ _ _ _]
                    tunnel: w302 -> [_ _ _ _ _ _ _ _ _ w635 _ _ _ _ _ _]
                    tunnel: w388 -> [_ _ _ _ _ _ _ _ _ _ _ _ _ w690 _ _]
                    tunnel: [w449 w464 w471 w478 w487 w498 w517 w534 w611 w632 w666 TRUE w682 w686 w699 w703] -> w298
                    tunnel: w384 -> [_ _ _ _ _ _ _ _ _ _ _ w668 _ _ _ _]
                    tunnel: w339 -> [_ _ _ _ w492 _ _ _ _ _ _ _ _ _ _ _]
                    tunnel: w337 -> [_ _ _ _ _ _ _ _ _ _ w656 _ _ _ _ _]
                    tunnel: w300 -> [_ _ _ _ _ _ _ w529 _ w624 _ _ _ _ _ w707]
                    frame "idle", Default {
                      w449 = FALSE
                      n238 = local read "trialStart"() -> (w450:bool)
                      n239 = case shown="True" w450 {
                        tunnel: [w453 w456] -> w451
                        tunnel: w448 -> [w453 _]
                        tunnel: w445 -> [w452 w455]
                        tunnel: [w452 w454] -> w446
                        frame False {
                        }
                        frame True {
                          n240 = stacked-sequence {
                            tunnel: [w457 _] -> w456
                            tunnel: w455 -> [_ w462]
                            tunnel: [_ w461] -> w454
                            frame #0 {
                              n241 = local read "toneReward"() -> (w458:bool)
                              n242 = case shown="False" w458 {
                                tunnel: [states_def."tone" states_def."vs before"] -> w457
                                frame True {
                                }
                                frame False {
                                }
                              }
                            }
                            frame #1 {
                              n243 = local write "trialStart"(FALSE) -> ()
                              n244 = Increment(x=w462) -> (x+1=w461:i32)
                            }
                          }
                        }
                      }
                    }
                    frame "vs before" {
                      w464 = FALSE
                      n245 = Select(t=states_def."vs", s=w470, f=w468) -> (s? t:f=w469:T5)
                    }
                    frame "vs" {
                      w471 = FALSE
                      n246 = Select(t=w476, s=w477, f=states_def."delay") -> (s? t:f=w475:T5)
                    }
                    frame "vs after" {
                      w478 = FALSE
                      n247 = Select(t=w484, s=w483, f=states_def."delay") -> (s? t:f=w482:T5)
                    }
                    frame "delay" {
                      w487 = FALSE
                      n248 = Not Equal?(x=w491, y=w490) -> (x != y?=w489:bool)
                      n249 = Select(t=w493, s=w489, f=w486) -> (s? t:f=w488:u64)
                      n250 = Add(x=w492, y=w488) -> (x+y=w494:u64)
                      n251 = Less?(x=w494, y=w493) -> (x < y?=w485:bool)
                      n252 = Select(t=states_def."tone after", s=w485, f=w490) -> (s? t:f=w497:T5)
                    }
                    frame "tone before" {
                      w498 = FALSE
                      n253 = case shown="True" w504 {
                        tunnel: [w509 states_def."tone after"] -> w500
                        tunnel: w506 -> [w509 _]
                        tunnel: w505 -> [w508 _]
                        tunnel: [w508 w512] -> w503
                        tunnel: w501 -> [_ w512]
                        tunnel: [TRUE FALSE] -> w499
                        frame False {
                        }
                        frame True {
                        }
                      }
                    }
                    frame "tone" {
                      w517 = FALSE
                      n254 = local read "Busy"() -> (w513:bool)
                      n255 = case shown="True" w513 {
                        tunnel: [w522 states_def."tone after"] -> w520
                        tunnel: w519 -> [w522 _]
                        tunnel: w515 -> [_ w523]
                        tunnel: [w521 w523] -> w516
                        tunnel: w514 -> [w521 _]
                        frame False {
                        }
                        frame True {
                        }
                      }
                    }
                    frame "tone after" {
                      w534 = FALSE
                      n256 = local read "toneReward"() -> (w531:bool)
                      n257 = local read "allowAutoWater"() -> (w527:bool)
                      n258 = Or(x=w531, y=w532) -> (x .or. y?=w530:bool)
                      n259 = case shown="True" w536 {
                        tunnel: w540 -> [_ w568]
                        tunnel: w539 -> [_ w567]
                        tunnel: w530 -> [_ w566]
                        tunnel: w529 -> [_ w565]
                        tunnel: [w557 w562] -> w526
                        tunnel: w528 -> [w557 w560]
                        frame False {
                        }
                        frame True {
                          n260 = case shown="True" w566 {
                            tunnel: [w584 w598] -> w563
                            tunnel: w568 -> [w581 w597]
                            tunnel: w567 -> [w585 w596]
                            tunnel: w565 -> [_ w595]
                            frame True {
                              n261 = Not(x=w581) -> (.not. x?=w586:bool)
                              n262 = Not(x=w585) -> (.not. x?=w582:bool)
                              n263 = local read "rightcounter"() -> (w578:i32)
                              n264 = local read "leftcounter"() -> (w579:i32)
                              n265 = Select(t=3, s="forceLRswitch", f=inf) -> (s? t:f=w569:dbl)
                              n266 = Select(t=3, s="forceLRswitch", f=inf) -> (s? t:f=w575:dbl)
                              n267 = Less?(x=w578, y=w569) -> (x < y?=w577:bool)
                              n268 = Compound Arithmetic op=AND(w586, w585, w577) -> (w583:bool)
                              n269 = Less?(x=w579, y=w575) -> (x < y?=w580:bool)
                              n270 = Compound Arithmetic op=AND(w580, w581, w582) -> (w576:bool)
                              n271 = case shown="True" w576 {
                                frame False {
                                }
                                frame True {
                                n272 = local read "leftcounter"() -> (w592:i32)
                                n273 = local write "FlagWaterLeft"(TRUE) -> ()
                                n274 = Increment(x=w592) -> (x+1=w593:i32)
                                n275 = local write "leftcounter"(w593) -> ()
                                n276 = local write "rightcounter"(0) -> ()
                                }
                              }
                              n277 = case shown="True" w583 {
                                frame False {
                                }
                                frame True {
                                n278 = local read "rightcounter"() -> (w588:i32)
                                n279 = local write "FlagWaterLeft"(FALSE) -> ()
                                n280 = Increment(x=w588) -> (x+1=w587:i32)
                                n281 = local write "rightcounter"(w587) -> ()
                                n282 = local write "leftcounter"(0) -> ()
                                }
                              }
                              n283 = Exclusive Or(1:w583, 2:w576) -> (0:w584:bool)
                            }
                            frame False {
                              # "Consider add another state for automaticaly give water \nwhen animal did not get water for consecutively 10 trials?"
                              n284 = case shown="2" w595 {
                                tunnel: [w601 w603] -> w598
                                tunnel: w597 -> [w600 w606]
                                tunnel: w596 -> [w599 w604]
                                frame 1, Default {
                                # "left"
                                n285 = Not(x=w599) -> (.not. x?=w602:bool)
                                n286 = And(x=w600, y=w602) -> (x .and. y?=w601:bool)
                                }
                                frame 2 {
                                # "right"
                                n287 = Not(x=w606) -> (.not. x?=w605:bool)
                                n288 = And(x=w605, y=w604) -> (x .and. y?=w603:bool)
                                }
                              }
                            }
                          }
                          n289 = local read "allowCorrection"() -> (w559:bool)
                          n290 = Select(t=w560, s=w559, f=states_def."timeout") -> (s? t:f=w558:T5)
                          n291 = Select(t=states_def."reward", s=w563, f=w558) -> (s? t:f=w562:T5)
                        }
                      }
                      n292 = case shown="True" w527 {
                        tunnel: w526 -> [w545 w555]
                        tunnel: [w545 w554] -> w525
                        frame False {
                        }
                        frame True {
                          w548 = 10 ("Priority")
                          n293 = local read "contNoReward"() -> (w552:i32)
                          n294 = Random Number (0-1)() -> (number: 0 to 1=w549:dbl)
                          n295 = Multiply(x=w549, y=w548) -> (x*y=w547:dbl)
                          n296 = Add(x=w547, y=w548) -> (x+y=w546:dbl)
                          n297 = Greater Or Equal?(x=w552, y=w546) -> (x >= y?=w551:bool)
                          n298 = Select(t=0 ("Priority"), s=w551, f=w552) -> (s? t:f=w550:i32)
                          n299 = Select(t=states_def."manualwater", s=w551, f=w555) -> (s? t:f=w554:T5)
                          n300 = local write "contNoReward"(w550) -> ()
                        }
                      }
                      n301 = Add(x=w535, y=w538) -> (x+y=w544:u64)
                      n302 = Greater?(x=w543, y=w544) -> (0:w541:bool)
                      n303 = Select(t=states_def."cycle end", s=w541, f=w525) -> (s? t:f=w542:T5)
                    }
                    frame "cycle end" {
                      w611 = FALSE
                      # "inform host computer to start \nanother trial"
                      n304 = case shown="False" w615 {
                        tunnel: [w616 w622] -> w612
                        tunnel: [states_def."idle" states_def."tone after"] -> w614
                        tunnel: w613 -> [w616 w622]
                        tunnel: [w617 w620] -> w608
                        tunnel: w610 -> [w617 w620]
                        tunnel: w609 -> [_ _]
                        tunnel: w607 -> [_ _]
                        frame False {
                          n305 = local write "trialDone"(TRUE) -> ()
                        }
                        frame True {
                        }
                      }
                    }
                    frame "reward" {
                      w632 = FALSE
                      n306 = Not Equal?(x=w644, y=w626) -> (x != y?=w639:bool)
                      n307 = local read "toneReward"() -> (w630:bool)
                      n308 = Select(t=w642, s=w639, f=w634) -> (s? t:f=w633:u64)
                      n309 = Or(x=w629, y=w630) -> (x .or. y?=w631:bool)
                      n310 = case shown="False" w631 {
                        tunnel: [w646 w649] -> w638
                        tunnel: [w645 w648] -> w637
                        tunnel: w624 -> [_ w647]
                        frame True {
                          n311 = local read "FlagWaterLeft"() -> (w646:bool)
                          n312 = Not(x=w646) -> (.not. x?=w645:bool)
                        }
                        frame False {
                          n313 = case shown="0, Default" w647 {
                            tunnel: [w650 w652 w653] -> w649
                            tunnel: [w650 w651 w654] -> w648
                            frame 0, Default {
                              w650 = FALSE
                            }
                            frame 1 {
                              w652 = TRUE
                              n314 = Not(x=w652) -> (.not. x?=w651:bool)
                            }
                            frame 2 {
                              w654 = TRUE
                              n315 = Not(x=w654) -> (.not. x?=w653:bool)
                            }
                          }
                        }
                      }
                      n316 = Add(x=w635, y=w633) -> (x+y=w643:u64)
                      n317 = Less?(x=w643, y=w642) -> (x < y?=w641:bool)
                      n318 = Select(t=states_def."reward refractory", s=w629, f=states_def."cycle end") -> (s? t:f=w625:T5)
                      n319 = local write "rewardStatus"(TRUE) -> ()
                      n320 = Select(t=w625, s=w641, f=w626) -> (s? t:f=w640:T5)
                    }
                    frame "reward refractory" {
                      w666 = FALSE
                      n321 = Not Equal?(x=w661, y=w661) -> (x != y?=w665:bool)
                      n322 = Select(t=w658, s=w665, f=w664) -> (s? t:f=w655:u64)
                      n323 = Add(x=w655, y=w656) -> (x+y=w657:u64)
                      n324 = Greater?(x=w658, y=w657) -> (0:w663:bool)
                      n325 = Select(t=states_def."cycle end", s=w663, f=w661) -> (s? t:f=w662:T5)
                    }
                    frame "punish" {
                      w667 = FALSE
                      n326 = Not Equal?(x=w675, y=w669) -> (x != y?=w677:bool)
                      n327 = case shown="True" w677 {
                        tunnel: w669 -> [_ w681]
                        frame False {
                        }
                        frame True {
                          "curState" <- w681
                        }
                      }
                      n328 = Select(t=w670, s=w677, f=w678) -> (s? t:f=w671:u64)
                      n329 = Add(x=w671, y=w668) -> (x+y=w672:u64)
                      n330 = Less?(x=w670, y=w672) -> (x < y?=w676:bool)
                      n331 = local read "curState"() -> (w674:u32)
                      n332 = Select(t=w669, s=w676, f=w674) -> (s? t:f=w673:u32)
                    }
                    frame "punish refractory" {
                      w682 = FALSE
                      # "To do"
                    }
                    frame "timeout" {
                      w686 = FALSE
                      # "To do: change the state when timeout finished?????"
                      n333 = Not Equal?(x=w695, y=w694) -> (x != y?=w698:bool)
                      n334 = Select(t=w692, s=w698, f=w691) -> (s? t:f=w689:u64)
                      n335 = Add(x=w689, y=w690) -> (x+y=w697:u64)
                      n336 = Greater?(x=w692, y=w697) -> (0:w696:bool)
                      n337 = Select(t=states_def."cycle end", s=w696, f=w694) -> (s? t:f=w693:T5)
                    }
                    frame "exit" {
                      w699 = FALSE
                    }
                    frame "manualwater" {
                      w703 = FALSE
                      n338 = case shown="1" w707 {
                        frame 0, Default {
                        }
                        frame 1 {
                          n339 = local write "manualWaterLeft"(TRUE) -> ()
                        }
                        frame 2 {
                          n340 = local write "manualWaterRight"(TRUE) -> ()
                        }
                      }
                    }
                  }
                  n341 = local read "rtFIFOdataPool"() -> (w345:u32)
                  n342 = local read "rtFIFOdataDim"() -> (w352:i32)
                  n343 = Multiply(x=w352, y=w345) -> (x*y=w353:u32)
                  n344 = local read "manualWaterRight"() -> (w306:bool)
                  n345 = case shown="False" w306 {
                    tunnel: [w408 w417] -> w304
                    tunnel: w305 -> [w409 _]
                    tunnel: w303 -> [w407 w417]
                    tunnel: w302 -> [w406 _]
                    frame False {
                      n346 = local read "rightWaterOnFlag"() -> (w405:bool)
                      n347 = case shown="True" w405 {
                        tunnel: w409 -> [_ w414]
                        tunnel: [0 w414] -> w408
                        tunnel: w407 -> [_ w416]
                        tunnel: w406 -> [_ w415]
                        frame False {
                        }
                        frame True {
                          n348 = Add(x=w415, y=w414) -> (x+y=w413:u64)
                          n349 = Greater?(x=w416, y=w413) -> (0:w412:bool)
                          n350 = Not(x=w412) -> (.not. x?=w411:bool)
                          n351 = local write "rightWaterOnFlag"(w411) -> ()
                        }
                      }
                    }
                    frame True {
                      n352 = local write "manualWaterRight"(FALSE) -> ()
                      n353 = local write "rightWaterOnFlag"(TRUE) -> ()
                    }
                  }
                  n354 = shared-variable ".\\variables - network - RT (separate).lvlib\\stop - network"() -> (w402:bool)  [unwired: 1 in, 1 out]
                  n355 = local read "leftWaterOnFlag"() -> (w307:bool)
                  n356 = local read "rightWaterOnFlag"() -> (w301:bool)
                  n357 = local read "manualShock"() -> (w351:bool)
                  n358 = local read "allowPunish"() -> (w350:bool)
                  n359 = call "punish_check.vi"("input state"=w392, "lick"=w366, "allow punish"=w350) -> ("punish"=w391:bool)
                  n360 = Select(t=states_def."exit", s=w402, f=w391) -> (s? t:f=w390:T5)
                  n361 = feedback-in #2(w390) -> ()
                  n362 = feedback-in #3(w390) -> ()
                  n363 = Or(x=w307, y=w370) -> (x .or. y?=w369:bool)
                  n364 = Or(x=w301, y=w368) -> (x .or. y?=w367:bool)
                  n365 = Or(x=w351, y=w298) -> (x .or. y?=w387:bool)
                  n366 = local read "ABORT"() -> (w331:bool)
                  n367 = Build Array(w371, w369, w367, w387) -> (w362:bool[])
                  n368 = Build Array (concatenate)(w365, w362, w364) -> (w363:bool[])
                  n369 = Boolean Array To Number(Boolean array=w363) -> (number=w313:u32)
                  n370 = Build Array (concatenate)(w356, w313, w311) -> (w354:dbl[])
                  n371 = Array Size(array=w354) -> (size(s)=w333:i32)
                  n372 = Build Array (concatenate)(w377, w354) -> (w375:dbl[])
                  n373 = local write "rtFIFOdataDim"(w333) -> ()
                  n374 = Array Size(array=w375) -> (size(s)=w372:i32)
                  n375 = Equal?(x=w372, y=w353) -> (x = y?=w374:bool)
                  n376 = Not Equal?(x=w333, y=9) -> (x != y?=w332:bool)
                  n377 = case shown="True" w374 {
                    tunnel: [w437 w444] -> w373
                    tunnel: w375 -> [w438 w441]
                    tunnel: [w438 sgl[] [] ("array type (2D Dbl)")] -> w376
                    tunnel: w347 -> [_ w440]
                    tunnel: w346 -> [w437 w439]
                    frame False {
                    }
                    frame True {
                      n378 = local read "rtFIFOtimeout"() -> (w442:u32)
                      n379 = RT FIFO Write(0:w440, 1:w441, 2:w442, 3:w439) -> (11:w444:errorcluster)  [unwired: 1 in, 3 out]
                    }
                  }
                  n380 = case shown="True" w332 {
                    frame False {
                    }
                    frame True {
                      n381 = One Button Dialog(message="The dimention of rtFIFOdata is not 4, pleae change the size of alocated network stream.") -> (true=w435:bool)  [unwired: 1 in]
                      n382 = local write "ABORT"(w435) -> ()
                    }
                  }
                  n383 = call-poly <vilib>:"DAQmx Write.vi"("task/channels in"=w336, "data"=w362, "error in"=w335) -> ("task out"=w396:refnum<k21>, "error out"=w395:errorcluster)  [unwired: 10 in, 1 out]
                  n384 = node-c288() -> ()  [unwired: 1 in, 1 out]
                }
                n385 = node-c288(5.0, 100 ("Priority")) -> (w230:T2)  [unwired: 1 in]
                n386 = timed-loop {
                  timing: w230 -> [_]
                  timing-out: [_] -> w229
                  tunnel: [w270] -> w207
                  tunnel: [w269] -> w206
                  tunnel: [w268] -> w209
                  tunnel: [w267] -> w208
                  tunnel: w228 -> [w266]
                  tunnel: w227 -> [w265]
                  tunnel: w214 -> [w264]
                  tunnel: w213 -> [w263]
                  shift-right: [w273] -> _
                  shift-left: w223 -> [w272]
                  stop <- w271 stop-if-true
                  n387 = node-c288() -> ()  [unwired: 1 in, 1 out]
                  n388 = property class="Network Stream Endpoint"(reference=w265, error in=w266) -> (reference out=w275:refnum<k21>, error out=w274:errorcluster, "Connected"=→"Is Connected":bool, "AvailElmntsForWrite"=→"Available Elements for Writing":i32)
                  n389 = RT FIFO Read(0:w264, 2:0, 3:w263) -> (8:w268:refnum<k33>, 9:w261:sgl[], 11:w267:errorcluster)  [unwired: 1 in, 2 out]
                  n390 = Empty Array?(array=w261) -> (empty?=w260:bool)
                  n391 = case shown="True" w260 {
                    tunnel: w261 -> [w283 _]
                    tunnel: [FALSE w288] -> w271
                    tunnel: w275 -> [w285 w286]
                    tunnel: w274 -> [w284 w287]
                    tunnel: [w278 w289] -> w273
                    tunnel: w272 -> [w281 w289]
                    tunnel: [w280 w286] -> w270
                    tunnel: [w279 w287] -> w269
                    frame False {
                      n392 = Increment(x=w281) -> (x+1=w278:i32)
                      n393 = shared-variable-write(w285, w284, w283) -> (w280:refnum<k21>, w279:errorcluster)  [unwired: 1 in, 1 out]
                      n394 = local write "stream counter"(w278) -> ()
                    }
                    frame True {
                      n395 = local read "ABORT"() -> (w288:bool)
                    }
                  }
                  n396 = node-c288() -> ()  [unwired: 1 in, 1 out]
                }
                n397 = node-c288(w229) -> (w197:errorcluster)
                n398 = node-c288(w233) -> (w199:errorcluster)
                n399 = Flush Stream(8:w206, 11:w207) -> (0:w205:errorcluster, 3:w204:refnum<k21>)  [unwired: 2 in, 1 out]
                n400 = RT FIFO Delete(0:w209, 3:w208) -> (11:w202:errorcluster)  [unwired: 1 in]
                n401 = Destroy Stream Endpoint(8:w205, 11:w204) -> (0:w203:errorcluster)
                n402 = node-c288(w231) -> (w198:errorcluster)
                n403 = stacked-sequence {
                  tunnel: w203 -> [w241]
                  tunnel: [w241] -> w196
                  frame #0 {
                    n404 = shared-variable "Sabrina-RT1\\variables - network - RT (separate).lvlib\\stop - network"(TRUE ("stop - network")) -> ()  [unwired: 1 in, 1 out]
                  }
                }
                n405 = Build Array(w194, w194, w194, w194) -> (w193:bool[])
                n406 = call-poly <vilib>:"DAQmx Write.vi"("task/channels in"=w201, "data"=w193, "error in"=w200) -> ("task out"=w174:refnum<k21>, "error out"=w173:errorcluster)  [unwired: 10 in, 1 out]
                n407 = call <vilib>:"DAQmx Stop Task.vi"("task/channels in"=w176, "error in"=w175) -> ("error out"=w172:errorcluster)  [unwired: 12 in, 1 out]
                n408 = call <vilib>:"DAQmx Stop Task.vi"("task/channels in"=w174, "error in"=w173) -> ("error out"=w171:errorcluster)  [unwired: 12 in, 1 out]
                n409 = Merge Errors(w191, w202) -> (w195:errorcluster)
                n410 = Merge Errors(w172, w171) -> (w177:errorcluster)
                n411 = Merge Errors(w199, w198, w197) -> (w178:errorcluster)
                n412 = Merge Errors(w178, w177, w195, w196) -> (w192:errorcluster)
                "error out" <- w192
                n413 = call <vilib>:"Simple Error Handler.vi"("error in (no error)"=w192) -> ()  [unwired: 4 in, 5 out]
              }
            }
          }
          frame #2 {
            n414 = Wait (ms)(milliseconds to wait=u32 100) -> ()  [unwired: 1 out]
          }
        }
      }
      n415 = UDP Close(connection ID=w23, 8:w22) -> (error out=w24:errorcluster)  [unwired: 1 out]
      n416 = UDP Close(connection ID=w18, 8:w19) -> (error out=w17:errorcluster)  [unwired: 1 out]
      n417 = call <vilib>:"Simple Error Handler.vi"("error in (no error)"=w24) -> ()  [unwired: 4 in, 5 out]
      n418 = call <vilib>:"Simple Error Handler.vi"("error in (no error)"=w17) -> ()  [unwired: 4 in, 5 out]
    }
  }
